vi "Control Process.vi"(2 "Firing Data":T2={"error"={"status"=FALSE, "code"=0, "source"=""}, "AngleMotorRefnum"={"DeviceStatus"={"status"=FALSE, "code"=0, "source"=""}, "Type"=enum."PWM", "PWM"={"PWM Channel"=enum."PWM 1", "DeadBand"={"Name"="", "maxPositivePwm"=0, "minPositivePwm"=0, "centerPwm"=0, "maxNegativePwm"=0, "minNegativePwm"=0, "angularRange"=0}}, "CAN"={"Device Number"=0, "Control Mode"=enum."Percent VBus", "Semaphore"=refnum, "Max Vout"=12.0, "TalonSRX Control Mode"=enum."Percent VBus"}, "Invert"=FALSE}, "LeftWheelRefnum"={"DeviceStatus"={"status"=FALSE, "code"=0, "source"=""}, "Type"=enum."PWM", "PWM"={"PWM Channel"=enum."Invalid", "DeadBand"={"Name"="", "maxPositivePwm"=0, "minPositivePwm"=0, "centerPwm"=0, "maxNegativePwm"=0, "minNegativePwm"=0, "angularRange"=0}}, "CAN"={"Device Number"=0, "Control Mode"=enum."Percent VBus", "Semaphore"=refnum, "Max Vout"=12.0, "TalonSRX Control Mode"=enum."Percent VBus"}, "Invert"=FALSE}, "RightWheelRefnum"={"DeviceStatus"={"status"=FALSE, "code"=0, "source"=""}, "Type"=enum."PWM", "PWM"={"PWM Channel"=enum."Invalid", "DeadBand"={"Name"="", "maxPositivePwm"=0, "minPositivePwm"=0, "centerPwm"=0, "maxNegativePwm"=0, "minNegativePwm"=0, "angularRange"=0}}, "CAN"={"Device Number"=0, "Control Mode"=enum."Percent VBus", "Semaphore"=refnum, "Max Vout"=12.0, "TalonSRX Control Mode"=enum."Percent VBus"}, "Invert"=FALSE}, "PushSolenoidRefnum"={"DevStatus"={"status"=FALSE, "code"=0, "source"=""}, "Pneumatics Control Module"=0, "Forward Solenoid Channel"=enum."Invalid", "Reverse Solenoid Channel"=enum."Invalid"}, "AngleMotorPosition(t)"=0.0, "LaunchSpeed(t/100ms)"=0.0, "CollectSpeed(t/100ms)"=0.0, "AngleThreshold"=0.0, "ShotDuration(10ms)"=0}, 3 "Manual Control":T1={"Joystick"=0.0, "LowerButton"=FALSE, "Aimbot?"=TRUE}, 4 "CollectionTrigger":bool, 5 "SpinupTrigger":bool) -> (0 "Speed":dbl, 1 "Angle":dbl)   [LabVIEW 2015]
doc: "Processes data from driver station for use outside of firing."
uses:
  Bundle.ctl
  <vilib>/Rock Robotics/WPI/MotorControl/WPI_MotorControlDeviceRef.ctl
  <vilib>/Rock Robotics/WPI/MotorControl/WPI_MotorControlType.ctl
  <vilib>/Rock Robotics/SystemInterfaces/DIO/FPGA_DIOPWMChannel.ctl
  <vilib>/Rock Robotics/WPI/PWM/WPI_PWMDeadband.ctl
  <vilib>/Rock Robotics/WPI/CAN/Jaguar/SubVIs/WPI_CANJaguar_ControlMode.ctl
  <vilib>/Rock Robotics/WPI/CAN/TalonSRX/WPI_CANTalonSRX_APIControlMode.ctl
  <vilib>/Rock Robotics/WPI/Solenoid/WPI_SolenoidDevRef.ctl
  <vilib>/Rock Robotics/WPI/Solenoid/WPI_SolenoidChannel.ctl
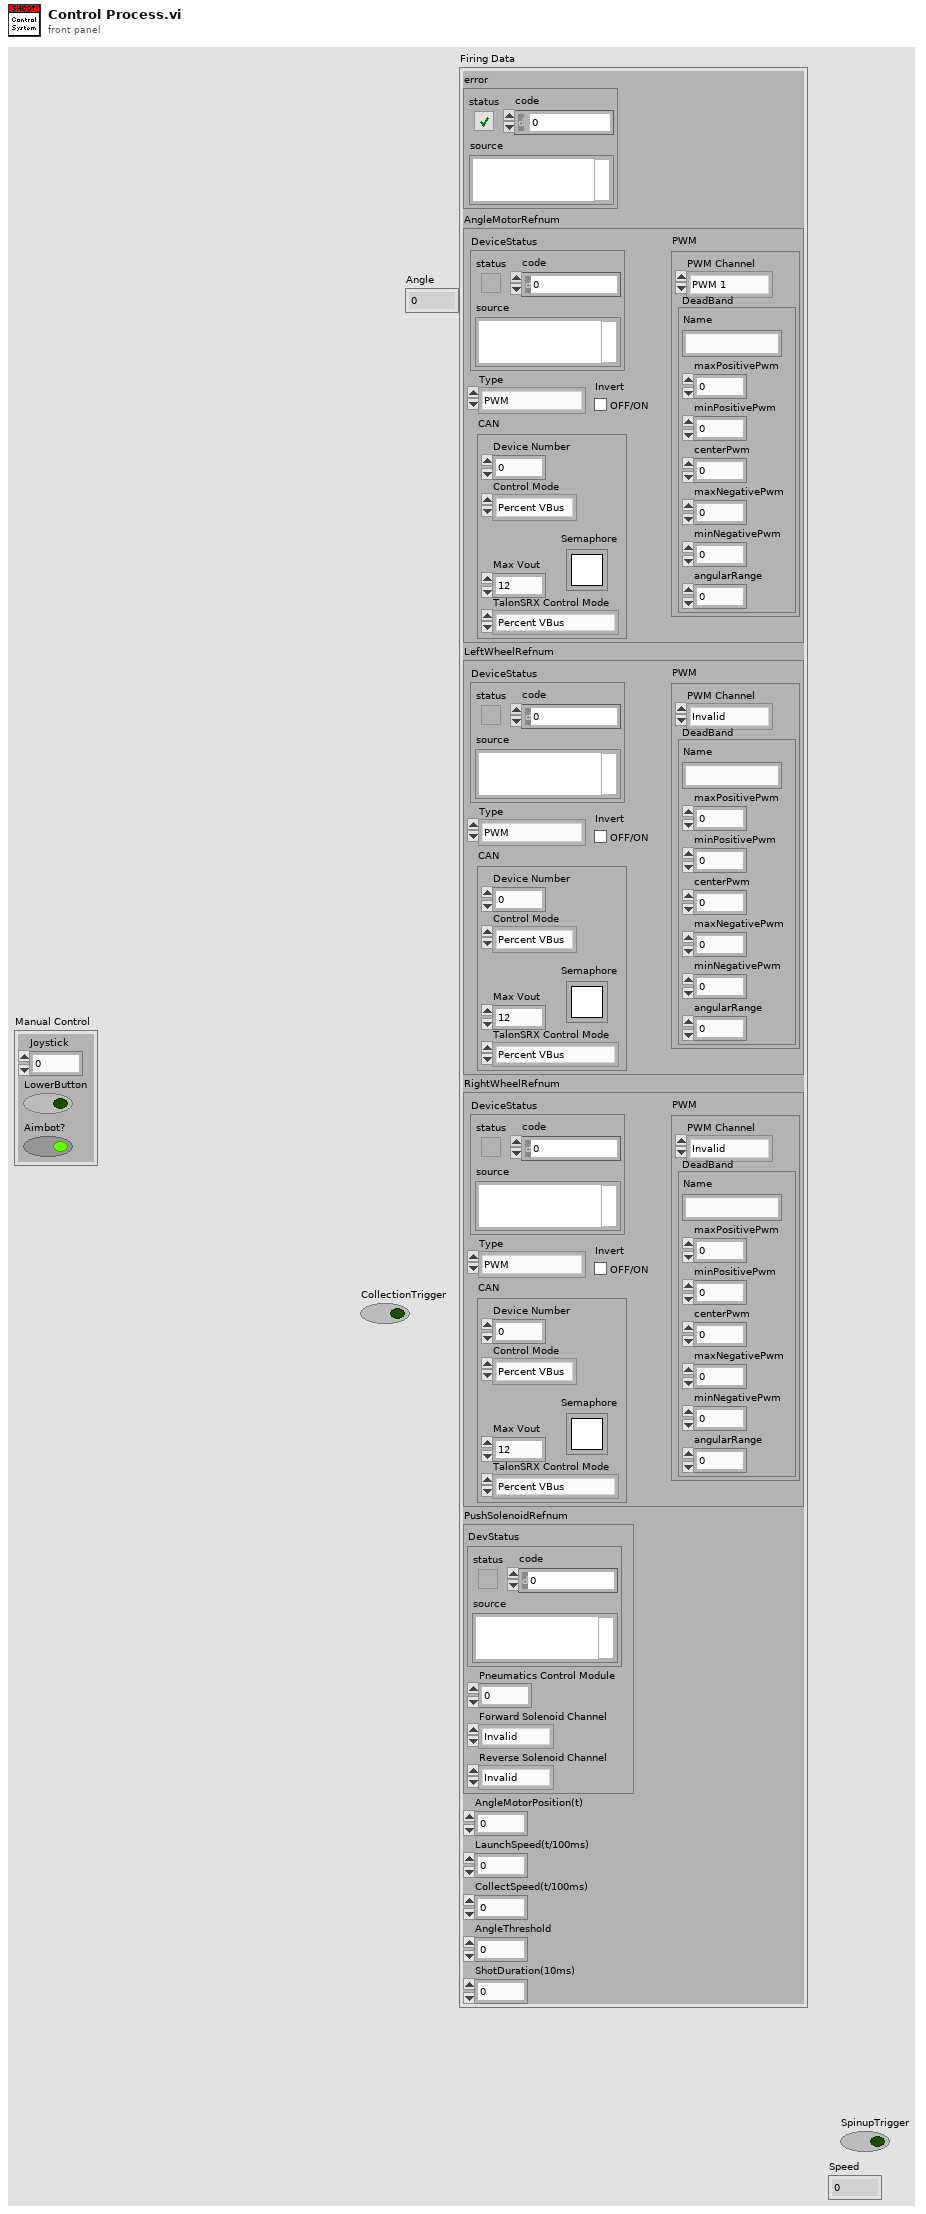
[diagram p1: front panel]
types:
  T1 = cluster{"Joystick":dbl, "LowerButton":bool, "Aimbot?":bool}
  T2 = typedef "Bundle.ctl" = cluster{"error":errorcluster, "AngleMotorRefnum":T3, "LeftWheelRefnum":T3, "RightWheelRefnum":T3, "PushSolenoidRefnum":T10, "AngleMotorPosition(t)":dbl, "LaunchSpeed(t/100ms)":dbl, "CollectSpeed(t/100ms)":dbl, "AngleThreshold":dbl, "ShotDuration(10ms)":i32}
  T3 = typedef "WPI_MotorControlDeviceRef.ctl" = cluster{"DeviceStatus":errorcluster, "Type":T4, "PWM":cluster{"PWM Channel":T5, "DeadBand":T6}, "CAN":cluster{"Device Number":u8, "Control Mode":T7, "Semaphore":T8, "Max Vout":dbl, "TalonSRX Control Mode":T9}, "Invert":bool}
  T4 = typedef "WPI_MotorControlType.ctl" = enum16{"PWM", "CAN", "CANTalonSRX"}
  T5 = typedef "FPGA_DIOPWMChannel.ctl" = enum8{"PWM 0", "PWM 1", "PWM 2", "PWM 3", "PWM 4", "PWM 5", "PWM 6", "PWM 7", "PWM 8", "PWM 9", "PWM MXP 0", "PWM MXP 1", "PWM MXP 2", "PWM MXP 3", "PWM MXP 4", "PWM MXP 5", "PWM MXP 6", "PWM MXP 7", "PWM MXP 8", "PWM MXP 9", "Invalid"}
  T6 = typedef "WPI_PWMDeadband.ctl" = cluster{"Name":string, "maxPositivePwm":i32, "minPositivePwm":i32, "centerPwm":i32, "maxNegativePwm":i32, "minNegativePwm":i32, "angularRange":u16}
  T7 = typedef "WPI_CANJaguar_ControlMode.ctl" = enum8{"Percent VBus", "Current", "Speed", "Position", "Voltage"}
  T8 = typedef "Semaphore RefNum" = refnum<k1>
  T9 = typedef "WPI_CANTalonSRX_APIControlMode.ctl" = enum8{"Percent VBus", "Speed", "Position", "Slave", "Unchanged / Invalid", "Voltage Compensation", "Current", "Motion Profile"}
  T10 = typedef "WPI_SolenoidDevRef.ctl" = cluster{"DevStatus":errorcluster, "Pneumatics Control Module":u8, "Forward Solenoid Channel":T11, "Reverse Solenoid Channel":T11}
  T11 = typedef "WPI_SolenoidChannel.ctl" = enum8{"Solenoid 0", "Solenoid 1", "Solenoid 2", "Solenoid 3", "Solenoid 4", "Solenoid 5", "Solenoid 6", "Solenoid 7", "Invalid"}
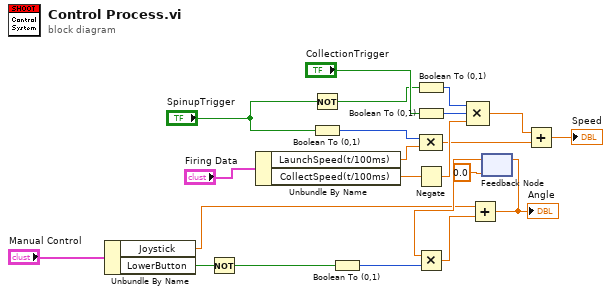
[diagram p0: block diagram]
diagram:
  n1 = Unbundle By Name("Manual Control") -> ("Joystick"=w1:dbl, "LowerButton"=w22:bool)
  n2 = Not(x=w22) -> (.not. x?=w20:bool)
  n3 = Unbundle By Name("Firing Data") -> ("LaunchSpeed(t/100ms)"=w11:dbl, "CollectSpeed(t/100ms)"=w13:dbl)
  n4 = Not(x="SpinupTrigger") -> (.not. x?=w14:bool)
  n5 = Boolean To (0,1)(Boolean="SpinupTrigger") -> (0, 1=w12:i16)
  n6 = Boolean To (0,1)(Boolean=w20) -> (0, 1=w21:i16)
  n7 = Boolean To (0,1)(Boolean=w14) -> (0, 1=w18:i16)
  n8 = Boolean To (0,1)(Boolean="CollectionTrigger") -> (0, 1=w17:i16)
  n9 = Negate(x=w13) -> (-x=w16:dbl)
  n10 = Compound Arithmetic op=MULTIPLY(w12, w11) -> (w9:dbl)
  n11 = Compound Arithmetic op=MULTIPLY(w18, w17, w16) -> (w8:dbl)
  n12 = feedback #1(0.0 ("t")) -> (w6:dbl)
  n13 = Multiply(x=w6, y=w21) -> (x*y=w2:dbl)
  n14 = Add(x=w1, y=w2) -> (x+y=w4:dbl)
  "Angle" <- w4
  n15 = feedback-in #1(w4) -> ()
  n16 = Add(x=w8, y=w9) -> (x+y=→"Speed":dbl)
